vi "Power-HWP test.vi"(8 "Error In":errorcluster, 10 "Cluster In":T2={"Position"=0.0, "Is.Enabled?"=FALSE, "Is.Connected?"=FALSE, "Device SN"="55151324", "AccelerationMaximum"=10.0, "VelocityMaximum"=10.0, "Acceleration"=10.0, "Velocity"=10.0, "waitTimeout (ms)"=10000, "Model"=enum."None", "Is.Homed?"=FALSE, "MOVE"=FALSE}) -> (0 "Error Out":errorcluster)   [LabVIEW 2018]
uses:
  Hardware Mfg/Thorlabs Translation Stages/Controls/Translation Stage Cluster.ctl
  General/Controls/Translation Stage Types.ctl
  C:/Project/SerialSectionOCT/SerialSectOCT/Labview Software/Thorlabs.MotionControl.Controls.dll
  Thorlabs.MotionControl.Controls.dll
  KnifeEdgeTestClt.ctl
  Hardware Mfg/Thorlabs Cage Rotation/refnum control.ctl
  General/Controls/Set Get Controls.ctl
  Hardware Mfg/Thorlabs Translation Stages/Controls/Motion Translation Module Control2.ctl
  <vilib>/DAQmx/read.llb/DAQmx Read (Analog 1D Wfm NChan NSamp).vi
  <vilib>/DAQmx/create/channels.llb/DAQmx Create Channel (AI-Voltage-Basic).vi
  <vilib>/DAQmx/configure/timing.llb/DAQmx Timing (Sample Clock).vi
  <vilib>/DAQmx/configure/task.llb/DAQmx Configure Logging (TDMS).vi
  <vilib>/DAQmx/configure/trigger.llb/DAQmx Start Trigger (Digital Edge).vi
  <vilib>/DAQmx/configure/trigger.llb/DAQmx Start Trigger (Time).vi
  <vilib>/DAQmx/configure/trigger.llb/DAQmx Start Trigger (Analog Edge).vi
  <vilib>/DAQmx/miscellaneous.llb/DAQmx Fill In Error Info.vi
  <resource>/objmgr/daqmx.rc
panel:
  in  "Trigger Type":T1(tab)
  in  "Digital Start Trigger Edge":i32(ring)=10280 caption="Edge" items=["Rising"=10280, "Falling"=10171]
  in  "Digital Start Trigger Source":tag="/Dev1/PFI0" caption="Source"
  in  "Digital Pause Trigger Pause When":i32(ring)=10192 caption="Pause When" items=["High"=10192, "Low"=10214]
  in  "Digital Pause Trigger Source":tag="/Dev1/PFI0" caption="Source"
  in  "Analog Start Trigger Level":dbl caption="Level" format="%0.2f"
  in  "Analog Start Trigger Hysteresis":dbl caption="Hysteresis" format="%.2f"
  in  "Analog Start Trigger Slope":i32(ring)=10280 caption="Slope" items=["Rising"=10280, "Falling"=10171]
  in  "Analog Start Trigger Source":string="APFI0" caption="Source"
  in  "Analog Pause Trigger Source":string="APFI0" caption="Source"
  in  "Analog Pause Trigger Pause When":i32(ring)=10093 caption="Pause When" items=["Above Level"=10093, "Below Level"=10107]
  in  "Analog Pause Trigger Level":dbl caption="Level" format="%.2f"
  in  "When":timestamp
  in  "Select Time\nManually":bool
  in  "Number of Samples":i32=100
  in  "TDMS File Path":path
  in  "Sample Rate":dbl=1000.0
  in  "Sample Clock Source":tag="OnboardClock"
  in  "Terminal Configuration":i32(ring)=-1 items=["default"=-1, "RSE"=10083, "NRSE"=10078, "Differential"=10106, "Pseudodifferential"=12529]
  in  "Max Voltage":dbl=5.0
  in  "Min Voltage":dbl=-5.0
  in  "Physical Channel":tag="Dev1/ai0"
  out "Actual Sample Rate":dbl=1000.0 format="%0.2f"
  in  "Logging Mode":i32(ring)=10231 items=["Off"=10231, "Log and Read"=15842]
  in  "LTS Reference":refnum<k24>(container)
  out "Power":dbl
  in  "Start":dbl
  in  "Stop":dbl=90.0
  in  "step size":dbl=1.0
  out "Wavelength [nm] 2":dbl caption="Wavelength"
  out "Avg. Time  [sec.]":dbl caption="Average Time"
  out "Average Count 2":i32 caption="Average Time"
  in  "Avg. Time (0.0) [sec.]":dbl=1.5 caption="Average Time (0.0)" min=0.1 max=5.0 step=0.1
  in  "Wavelength [nm]":dbl=840.0 caption="Wavelength (0.0)"
  in  "Average Count":i32=10 min=1 step=1
  in  "path":path=path "C:/Users/BOAS-USER/Documents/Data/210615_2P_power_calibration/test.csv"
  # "To enable triggers, select a tab above, and configure the settings.\n\nNot all hardware supports all trigger types. Refer to your device documentation for more information."
  # "This trigger type is not supported in continuous sample timing. \n\nRefer to your device documentation for more information on which triggers are supported."
  # "This trigger type is not supported in continuous sample timing. \n\nRefer to your device documentation for more information on which triggers are supported."
  # "If time is not manually set, task will begin after 10 seconds"
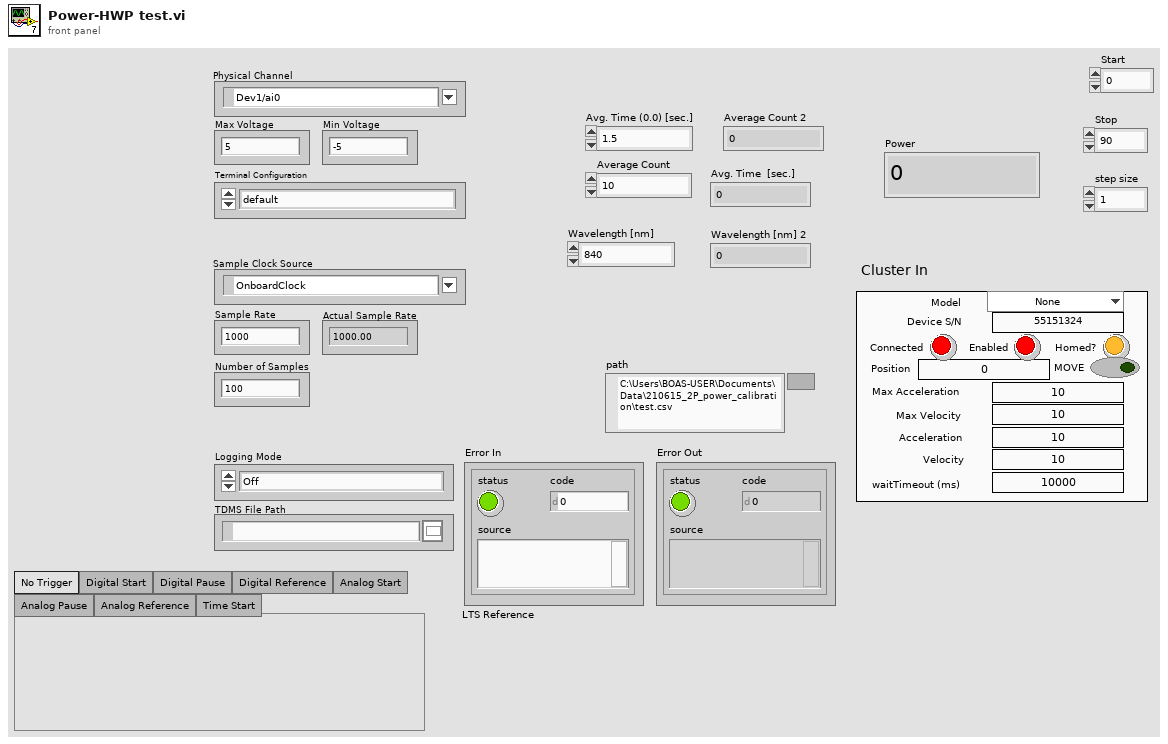
[diagram p1: front panel]
types:
  T1 = enum32{"No Trigger", "Digital Start", "Digital Pause", "Digital Reference", "Analog Start", "Analog Pause", "Analog Reference", "Time Start"}
  T2 = typedef "Translation Stage Cluster.ctl" = cluster{"Position":dbl, "Is.Enabled?":bool, "Is.Connected?":bool, "Device SN":string, "AccelerationMaximum":dbl, "VelocityMaximum":dbl, "Acceleration":dbl, "Velocity":dbl, "waitTimeout (ms)":i32, "Model":T3, "Is.Homed?":bool, "MOVE":bool}
  T3 = typedef "Translation Stage Types.ctl" = enum16{"None", "Thorlabs LTS", "Thorlabs MLJ"}
  T4 = typedef "KnifeEdgeTestClt.ctl" = enum16{"Init Power meter", "Init Table stages", "Go stage home", "Move stage", "Power meter thorlabs", "Uninit", "Generate steps", "Power meter PDA50B2", "Init PDA50B2"}
  T5 = typedef "refnum control.ctl" = enum16{"Get", "Init"}
  T6 = typedef "Motion Translation Module Control2.ctl" = enum16{"Init", "Home", "Status", "Velocity/Accel", "Position", "Jog", "Stop", "Uninit", "Enable", "Disable"}
  T7 = typedef "Set Get Controls.ctl" = enum16{"Set", "Get"}
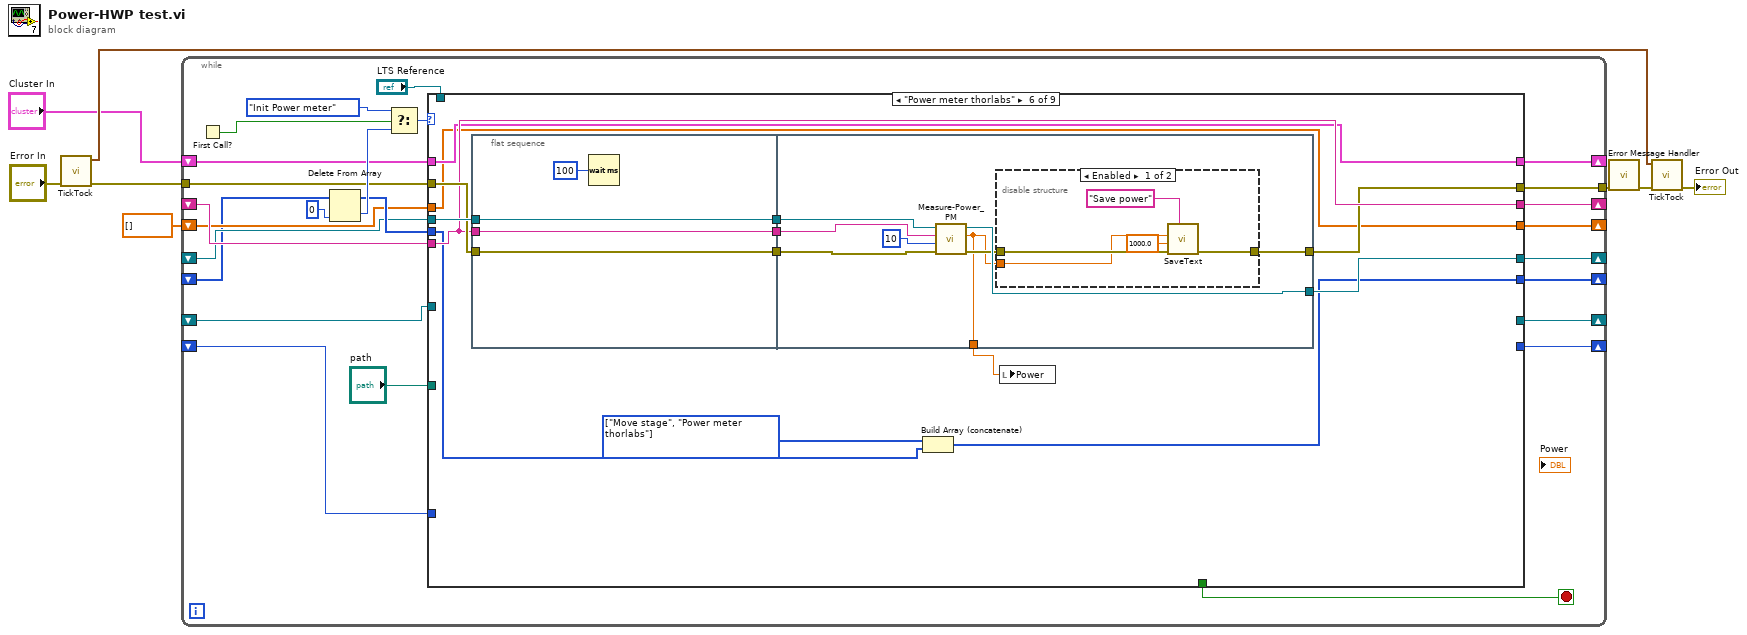
[diagram p0: block diagram]
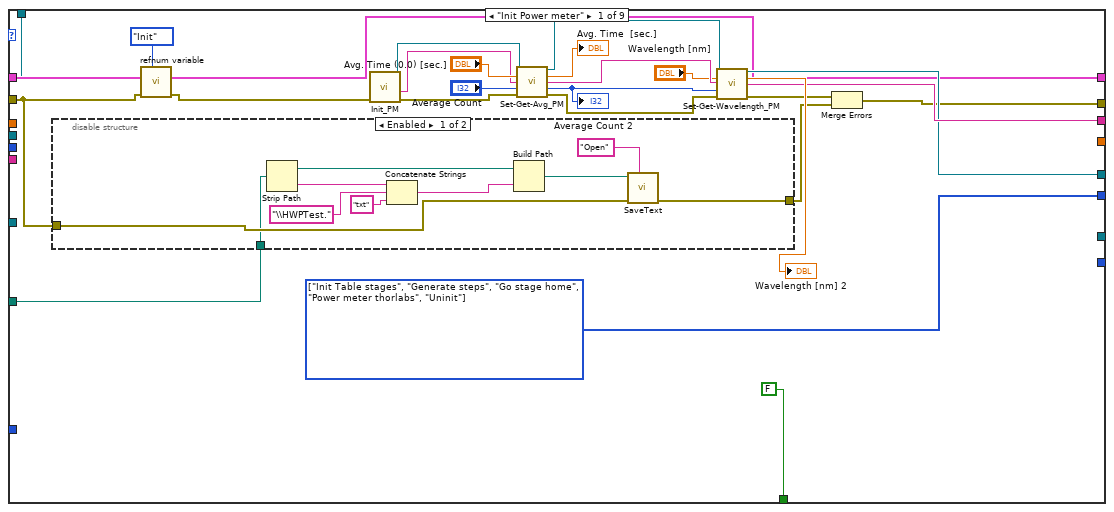
[diagram p2: hidden frame]
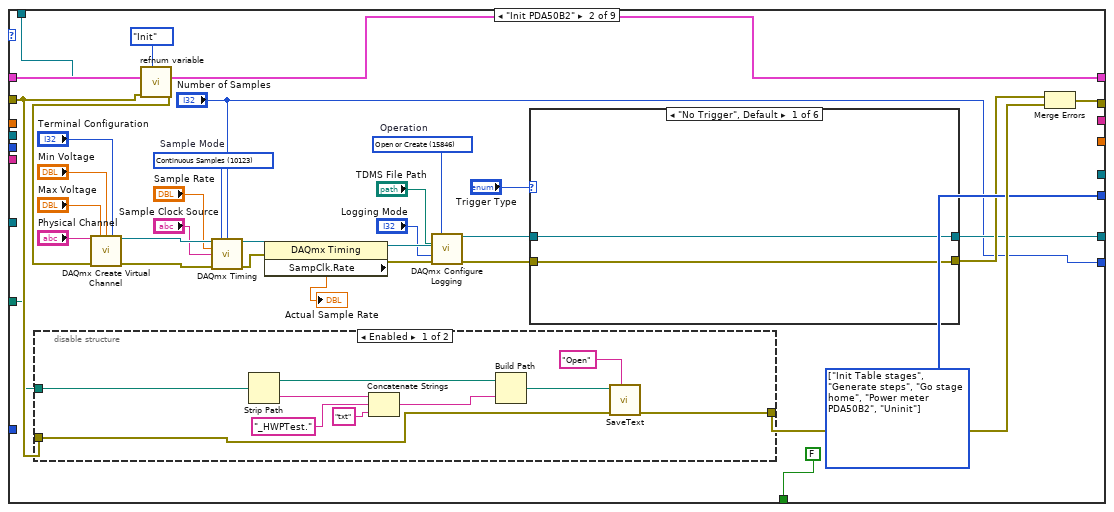
[diagram p4: hidden frame]
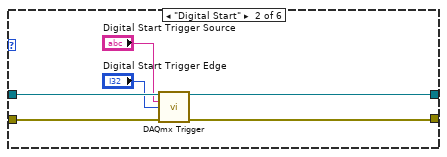
[diagram p5: hidden frame]
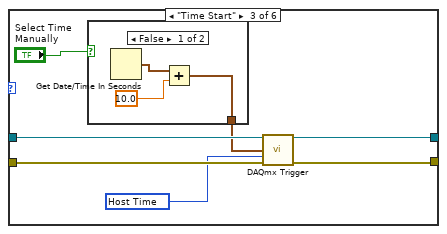
[diagram p6: hidden frame]
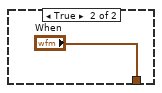
[diagram p7: hidden frame]
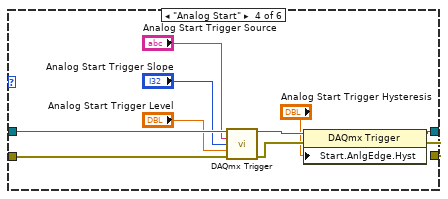
[diagram p8: hidden frame]
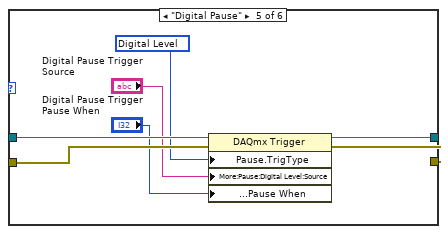
[diagram p9: hidden frame]
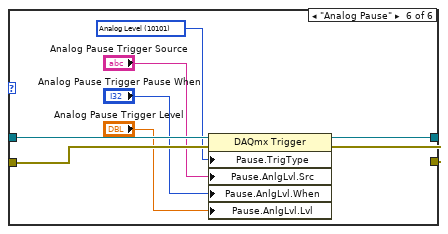
[diagram p10: hidden frame]
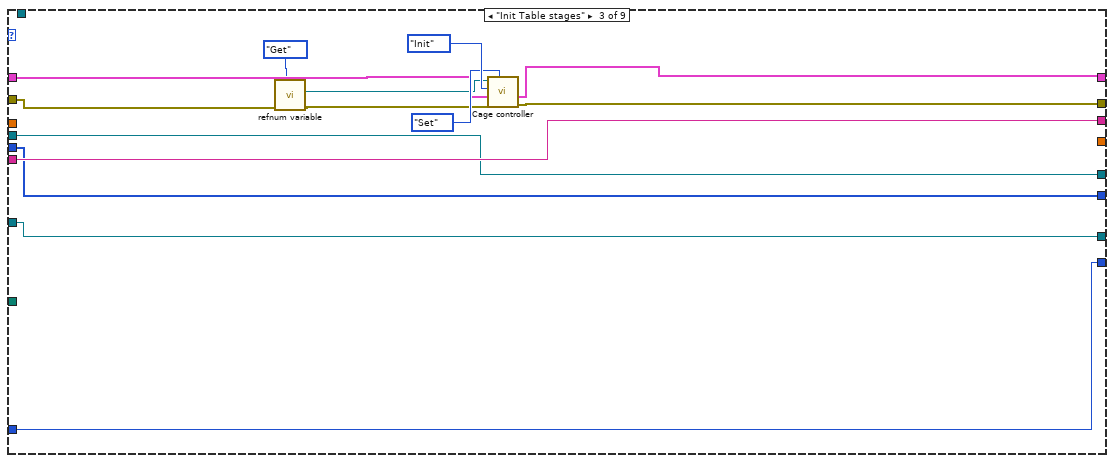
[diagram p12: hidden frame]
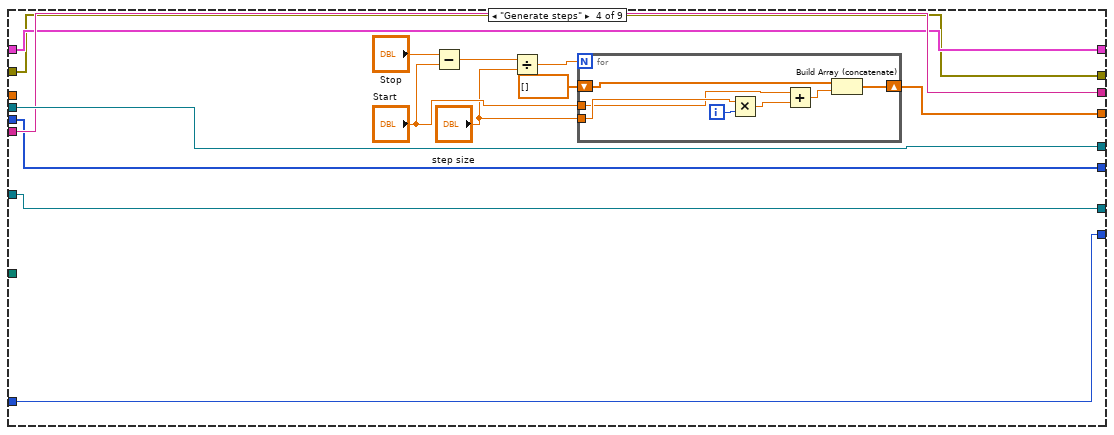
[diagram p13: hidden frame]
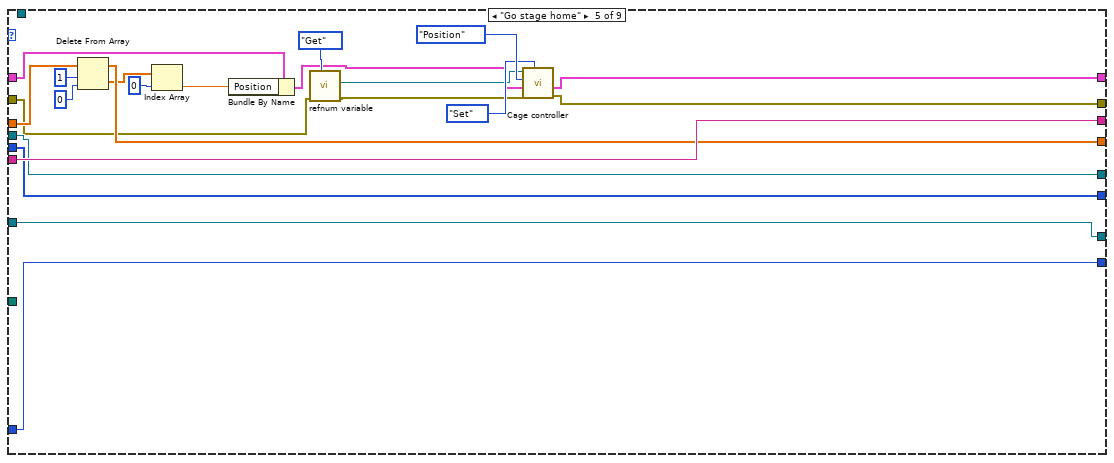
[diagram p14: hidden frame]
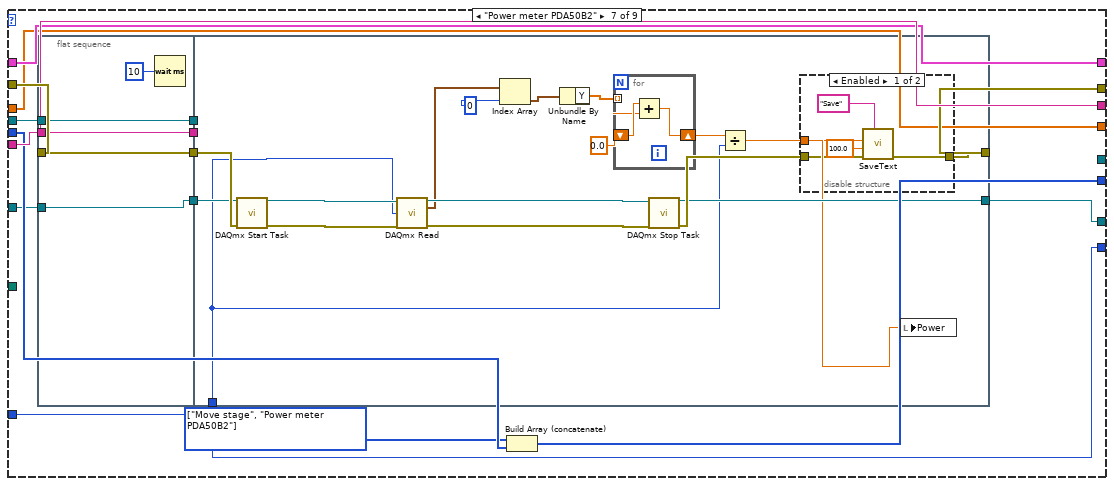
[diagram p16: hidden frame]
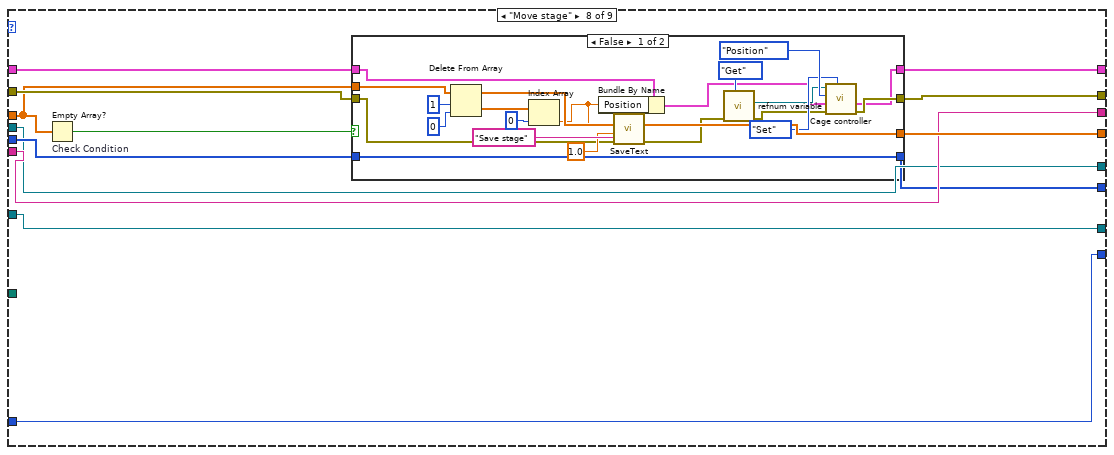
[diagram p18: hidden frame]
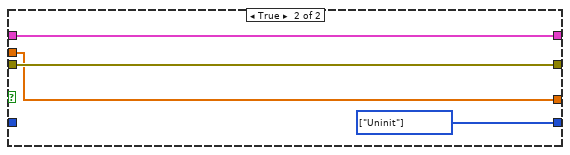
[diagram p19: hidden frame]
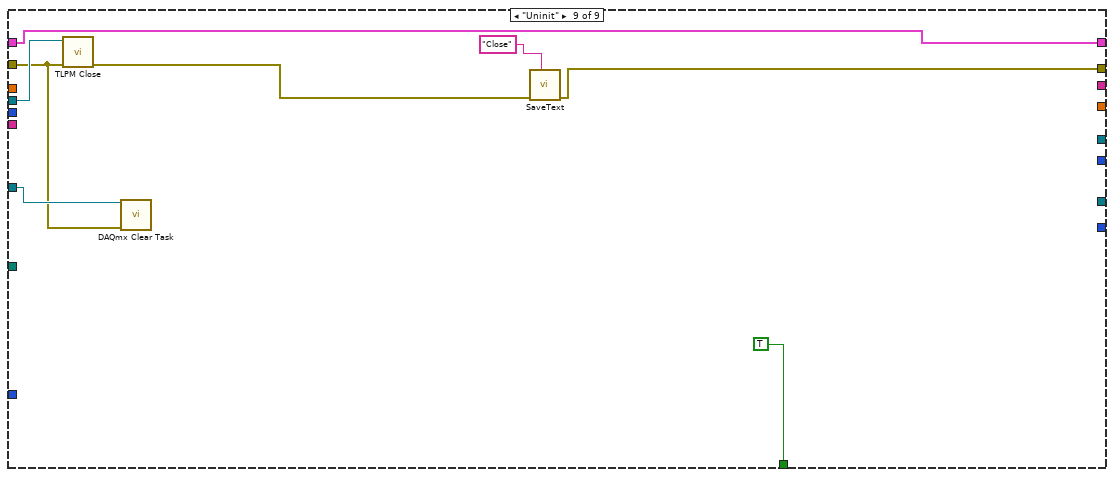
[diagram p20: hidden frame]
diagram:
  n1 = call "TickTock.vi"("Error In"="Error In") -> ("Error Out"=w6:errorcluster, "Current Time (Out)"=w4:timestamp)  [unwired: 8 in, 1 out]
  n2 = while {
    tunnel: w6 -> [w29]
    tunnel: [w28] -> w8
    shift-right: [w27] -> _
    shift-left: _ -> [w25]
    shift-right: [w26] -> _
    shift-left: _ -> [w24]
    shift-right: [w21] -> _
    shift-left: "Cluster In" -> [w22]
    shift-right: [w20] -> _
    shift-left: dbl[] [] -> [w19]
    shift-right: [w18] -> _
    shift-left: _ -> [w17]
    shift-right: [w14] -> _
    shift-left: _ -> [w11]
    shift-right: [w13] -> _
    shift-left: _ -> [w12]
    stop <- w16 stop-if-true
    n3 = First Call?() -> (First Call?: T/F=w15:bool)
    n4 = Delete From Array(array=w17, index=0) -> (deleted portion=w32:T4, array with subset deleted=w31:T4[])  [unwired: 1 in]
    n5 = Select(t=KnifeEdgeTestClt."Init Power meter", s=w15, f=w32) -> (s? t:f=w33:T4)
    n6 = case shown="\"Power meter thorlabs\"" w33 {
      tunnel: [w36 w95 w167 w175 w203 w215 w250 w295 _] -> w18
      tunnel: w31 -> [_ _ w167 w175 w203 w216 w251 w302 _]
      tunnel: [_ _ _ w171 w208 w217 w252 w304 _] -> w20
      tunnel: w29 -> [w39 w97 w160 w170 w196 w225 w259 w301 w330]
      tunnel: [w43 w100 w166 w170 w195 w222 w257 w300 w334] -> w28
      tunnel: [w46 _ w169 w182 w212 w223 w258 w299 _] -> w27
      tunnel: [w45 _ w168 w183 w202 w224 _ w298 _] -> w26
      tunnel: w25 -> [_ _ w169 w182 w212 w223 w258 w299 _]
      tunnel: w24 -> [_ _ w168 w183 w202 w226 w260 w298 w337]
      tunnel: w22 -> [w41 w99 w163 w181 w207 w218 w253 w297 w336]
      tunnel: [w41 w99 w162 w181 w193 w218 w253 w296 w336] -> w21
      tunnel: w19 -> [_ _ _ _ w211 w217 w252 w294 _]
      tunnel: [FALSE FALSE _ _ _ _ _ _ TRUE] -> w16
      tunnel: [_ w72 w157 w173 w192 _ w246 w293 _] -> w14
      tunnel: [_ "Number of Samples" w156 w172 w191 _ w245 w292 _] -> w13
      tunnel: w12 -> [_ _ w156 w172 w191 _ w245 w292 _]
      tunnel: w11 -> [_ _ w157 w173 w192 _ w247 w293 w332]
      tunnel: "path" -> [w35 w70 _ _ _ _ _ _ _]
      tunnel: "LTS Reference" -> [w34 w69 _ _ _ _ _ _ _]
      frame "Init Power meter" {
        w36 = T4[] [enum."Init Table stages", enum."Generate steps", enum."Go stage home", enum."Power meter thorlabs", enum."Uninit"] items=["Init Power meter", "Init Table stages", "Go stage home", "Move stage", "Power meter thorlabs", "Uninit", "Generate steps", "Power meter PDA50B2", "Init PDA50B2"]
        n7 = disable-structure shown="Enabled" {
          disable-tunnel: w39 -> [w64 _]
          disable-tunnel: [w63 _] -> w44
          disable-tunnel: w35 -> [w59 _]
          frame Enabled {
            n8 = Strip Path(path=w59) -> (stripped path=w61:path, name=w66:string)
            n9 = Concatenate Strings(w66, "\\HWPTest." ("string"), "txt" ("string")) -> (w62:string)
            n10 = Build Path(base path=w61, name or relative path=w62) -> (appended path=w60:path)
            n11 = call "SaveText.vi"("action"="Open", "error in"=w64, "file path (use dialog)"=w60) -> ("error out"=w63:errorcluster)  [unwired: 8 in]
          }
          frame Disabled {
          }
        }
        n12 = call "refnum variable.vi"("action"=refnum_control."Init", "error in (no error)"=w39, "reference in"=w34) -> ("error out"=w38:errorcluster)  [unwired: 7 in, 1 out]
        n13 = call "Init_PM.vi"("error in (no error)"=w38) -> ("error out"=w47:errorcluster, "Sensor Name"=w48:string, "instrument handle out"=w49:refnum<visa-resource-name>)  [unwired: 8 in]
        n14 = call "Set-Get-Avg_PM.vi"("instrument handle"=w49, "Average Time (0.0)"="Avg. Time (0.0) [sec.]", "Sensor"=w48, "Average Count"="Average Count", "error in (no error)"=w47) -> ("instrument handle out"=w56:refnum<visa-resource-name>, "Average Time"=→"Avg. Time  [sec.]":dbl, "Sensor 2"=w54:string, "Average Count"=w53:i32, "error out"=w57:errorcluster)  [unwired: 6 in]
        "Average Count 2" <- w53
        n15 = call "Set-Get-Wavelength_PM.vi"("instrument handle"=w56, "Wavelength"="Wavelength [nm]", "Sensor Name"=w54, "Average Count"=w53, "error in (no error)"=w57) -> ("instrument handle out"=w45:refnum<visa-resource-name>, "Wavelength"=→"Wavelength [nm] 2":dbl, "Sensor Name 2"=w46:string, "error out"=w42:errorcluster)  [unwired: 6 in, 1 out]
        n16 = Merge Errors(w42, w44) -> (w43:errorcluster)
      }
      frame "Init PDA50B2" {
        w87 = 15846 items=["Open"=10437, "Open or Create"=15846, "Create or Replace"=15847, "Create"=15848]  # Operation
        w92 = 10123 items=["Finite Samples"=10178, "Continuous Samples"=10123, "Hardware Timed Single Point"=12522]  # Sample Mode
        w95 = T4[] [enum."Init Table stages", enum."Generate steps", enum."Go stage home", enum."Power meter PDA50B2", enum."Uninit"] items=["Init Power meter", "Init Table stages", "Go stage home", "Move stage", "Power meter thorlabs", "Uninit", "Generate steps", "Power meter PDA50B2", "Init PDA50B2"]
        n17 = disable-structure shown="Enabled" {
          disable-tunnel: w97 -> [w151 _]
          disable-tunnel: [w150 _] -> w101
          disable-tunnel: w70 -> [w146 _]
          frame Enabled {
            n18 = Strip Path(path=w146) -> (stripped path=w148:path, name=w153:string)
            n19 = Concatenate Strings(w153, "_HWPTest." ("string"), "txt" ("string")) -> (w149:string)
            n20 = Build Path(base path=w148, name or relative path=w149) -> (appended path=w147:path)
            n21 = call "SaveText.vi"("action"="Open", "error in"=w151, "file path (use dialog)"=w147) -> ("error out"=w150:errorcluster)  [unwired: 8 in]
          }
          frame Disabled {
          }
        }
        n22 = call "refnum variable.vi"("action"=refnum_control."Init", "error in (no error)"=w97, "reference in"=w69) -> ("error out"=w73:errorcluster)  [unwired: 7 in, 1 out]
        n23 = call-poly <vilib>:"DAQmx Create Virtual Channel.vi"("maximum value"="Max Voltage", "minimum value"="Min Voltage", "input terminal configuration"="Terminal Configuration", "physical channels"="Physical Channel", "error in"=w73) -> ("task out"=w90:refnum<k21>, "error out"=w91:errorcluster)  [unwired: 9 in]
        n24 = call-poly <vilib>:"DAQmx Timing.vi"("task/channels in"=w90, "sample mode"=w92, "samples per channel"="Number of Samples", "rate"="Sample Rate", "source"="Sample Clock Source", "error in"=w91) -> ("task out"=w94:refnum<k21>, "error out"=w93:errorcluster)  [unwired: 8 in]
        n25 = property class="DAQmx Timing"(reference=w94, error in=w93) -> (reference out=w89:refnum<k21>, error out=w88:errorcluster, "SampClk.Rate"=→"Actual Sample Rate":dbl)
        n26 = call-poly <vilib>:"DAQmx Configure Logging.vi"("task/channels in"=w89, "operation"=w87, "file path"="TDMS File Path", "logging mode"="Logging Mode", "error in"=w88) -> ("task out"=w76:refnum<k21>, "error out"=w75:errorcluster)  [unwired: 9 in]
        n27 = case shown="\"No Trigger\", Default" "Trigger Type" {
          tunnel: w76 -> [w103 w109 w116 w130 w137 w145]
          tunnel: w75 -> [w102 w108 w115 w129 w134 w142]
          tunnel: [w103 w107 w114 w127 w136 w144] -> w72
          tunnel: [w102 w106 w113 w126 w135 w143] -> w74
          frame "No Trigger", Default {
          }
          frame "Digital Start" {
            n28 = call-poly <vilib>:"DAQmx Trigger.vi"("task/channels in"=w109, "source"="Digital Start Trigger Source", "edge"="Digital Start Trigger Edge", "error in"=w108) -> ("task out"=w107:refnum<k21>, "error out"=w106:errorcluster)  [unwired: 10 in]
          }
          frame "Time Start" {
            w112 = 16126 items=["Host Time"=16126, "I/O Device Time"=16127] ("timescale")
            n29 = case shown="False" "Select Time\nManually" {
              tunnel: [w117 "When"] -> w110
              frame False {
                n30 = Get Date/Time In Seconds() -> (seconds since 1Jan1904=w119:timestamp)
                n31 = Add(x=w119, y=10.0) -> (x+y=w117:timestamp)
              }
              frame True {
              }
            }
            n32 = call-poly <vilib>:"DAQmx Trigger.vi"("task/channels in"=w116, "when"=w110, "timescale"=w112, "error in"=w115) -> ("task out"=w114:refnum<k21>, "error out"=w113:errorcluster)  [unwired: 10 in]
          }
          frame "Analog Start" {
            n33 = call-poly <vilib>:"DAQmx Trigger.vi"("task/channels in"=w130, "source"="Analog Start Trigger Source", "slope"="Analog Start Trigger Slope", "level"="Analog Start Trigger Level", "error in"=w129) -> ("task out"=w125:refnum<k21>, "error out"=w124:errorcluster)  [unwired: 9 in]
            n34 = property class="DAQmx Trigger"(reference=w125, error in=w124, "Start.AnlgEdge.Hyst"="Analog Start Trigger Hysteresis") -> (reference out=w127:refnum<k21>, error out=w126:errorcluster)
          }
          frame "Digital Pause" {
            w133 = 10152 items=["Analog Level"=10101, "Analog Window"=10103, "Digital Level"=10152, "Digital Pattern"=10398, "None"=10230] ("Pause.TrigType")
            n35 = property class="DAQmx Trigger"(reference=w137, error in=w134, "Pause.TrigType"=w133, "More:Pause:Digital Level:Source"="Digital Pause Trigger Source", "More:Pause:Digital Level:Pause When"="Digital Pause Trigger Pause When") -> (reference out=w136:refnum<k21>, error out=w135:errorcluster)
          }
          frame "Analog Pause" {
            w141 = 10101 items=["Analog Level"=10101, "Analog Window"=10103, "Digital Level"=10152, "Digital Pattern"=10398, "None"=10230] ("Pause.TrigType")
            n36 = property class="DAQmx Trigger"(reference=w145, error in=w142, "Pause.TrigType"=w141, "Pause.AnlgLvl.Src"="Analog Pause Trigger Source", "Pause.AnlgLvl.When"="Analog Pause Trigger Pause When", "Pause.AnlgLvl.Lvl"="Analog Pause Trigger Level") -> (reference out=w144:refnum<k21>, error out=w143:errorcluster)
          }
        }
        n37 = Merge Errors(w74, w101) -> (w100:errorcluster)
      }
      frame "Init Table stages" {
        n38 = call "refnum variable.vi"("action"=refnum_control."Get", "error in (no error)"=w160) -> ("error out"=w159:errorcluster, "reference in 2"=w158:refnum<k24>)  [unwired: 8 in]
        n39 = call "Cage controller.vi"("Set/Get"=Set_Get_Controls."Set", "error in (no error)"=w159, "Cluster In"=w163, "Action"=Motion_Translation_Module_Control2."Init", "reference in"=w158) -> ("error out"=w166:errorcluster, "Cluster out"=w162:T2)  [unwired: 4 in, 1 out]
      }
      frame "Generate steps" {
        n40 = Subtract(x="Stop", y="Start") -> (x-y=w179:dbl)
        n41 = Divide(x=w179, y="step size") -> (x/y=w178:dbl)
        n42 = for {
          N: w178 -> [_]
          tunnel: "Start" -> [w188]
          tunnel: "step size" -> [w189]
          shift-right: [w185] -> w171
          shift-left: dbl[] [] -> [w184]
          i -> [w190]
          n43 = Multiply(x=w189, y=w190) -> (x*y=w187:dbl)
          n44 = Add(x=w188, y=w187) -> (x+y=w186:dbl)
          n45 = Build Array (concatenate)(w184, w186) -> (w185:dbl[])
        }
      }
      frame "Go stage home" {
        n46 = Delete From Array(array=w211, length=1, index=0) -> (deleted portion=w206:dbl[], array with subset deleted=w208:dbl[])
        n47 = Index Array(array=w206, index=0) -> (element=w204:dbl)
        n48 = Bundle By Name(cluster=w207, "Position"=w204) -> (w194:T2)
        n49 = call "refnum variable.vi"("action"=refnum_control."Get", "error in (no error)"=w196) -> ("error out"=w198:errorcluster, "reference in 2"=w197:refnum<k24>)  [unwired: 8 in]
        n50 = call "Cage controller.vi"("Set/Get"=Set_Get_Controls."Set", "error in (no error)"=w198, "Cluster In"=w194, "Action"=Motion_Translation_Module_Control2."Position", "reference in"=w197) -> ("error out"=w195:errorcluster, "Cluster out"=w193:T2)  [unwired: 4 in, 1 out]
      }
      frame "Power meter thorlabs" {
        w214 = T4[] [enum."Move stage", enum."Power meter thorlabs"] items=["Init Power meter", "Init Table stages", "Go stage home", "Move stage", "Power meter thorlabs", "Uninit", "Generate steps", "Power meter PDA50B2", "Init PDA50B2"]
        n51 = flat-sequence {
          tunnel: w223 -> [w228]
          tunnel: w225 -> [w229]
          tunnel: w226 -> [w230]
          tunnel: [w230] -> w221
          tunnel: [w229] -> w220
          tunnel: [w228] -> w219
          tunnel: [w236] -> w224
          tunnel: [w234] -> w222
          tunnel: w221 -> [w238]
          tunnel: w220 -> [w237]
          tunnel: w219 -> [w235]
          tunnel: [w231] -> w213
          frame #0 {
            n52 = Wait (ms)(milliseconds to wait=u32 100) -> ()  [unwired: 1 out]
          }
          frame #1 {
            n53 = call "Measure-Power_PM.vi"("error in (no error)"=w237, "Numeric"=10, "Sensor"=w235, "instrument handle"=w238) -> ("error out"=w232:errorcluster, "Power"=w231:dbl, "instrument handle out"=w236:refnum<visa-resource-name>)  [unwired: 5 in]
            n54 = disable-structure shown="Enabled" {
              disable-tunnel: [w243 w244] -> w234
              disable-tunnel: w232 -> [w242 w244]
              disable-tunnel: w231 -> [w240 _]
              frame Enabled {
                n55 = call "SaveText.vi"("action"="Save power", "error in"=w242, "GAIN"=sgl 1000.0, "data in"=w240) -> ("error out"=w243:errorcluster)  [unwired: 7 in]
              }
              frame Disabled {
              }
            }
          }
        }
        n56 = Build Array (concatenate)(w214, w216) -> (w215:T4[])
        n57 = local write "Power"(w213) -> ()
      }
      frame "Power meter PDA50B2" {
        w249 = T4[] [enum."Move stage", enum."Power meter PDA50B2"] items=["Init Power meter", "Init Table stages", "Go stage home", "Move stage", "Power meter thorlabs", "Uninit", "Generate steps", "Power meter PDA50B2", "Init PDA50B2"]
        n58 = flat-sequence {
          tunnel: w258 -> [w263]
          tunnel: w259 -> [w264]
          tunnel: w260 -> [w265]
          tunnel: [w265] -> w256
          tunnel: [w264] -> w255
          tunnel: [w263] -> w254
          tunnel: w247 -> [w261]
          tunnel: [w261] -> w248
          tunnel: [w282] -> w257
          tunnel: w256 -> [_]
          tunnel: w255 -> [w277]
          tunnel: w254 -> [_]
          tunnel: w245 -> [w271]
          tunnel: w248 -> [w275]
          tunnel: [w274] -> w246
          frame #0 {
            n59 = Wait (ms)(milliseconds to wait=u32 10) -> ()  [unwired: 1 out]
          }
          frame #1 {
            n60 = call <vilib>:"DAQmx Start Task.vi"("task/channels in"=w275, "error in"=w277) -> ("task out"=w281:refnum<k21>, "error out"=w280:errorcluster)  [unwired: 12 in]
            n61 = call-poly <vilib>:"DAQmx Read.vi"("task/channels in"=w281, "number of samples per channel"=w271, "error in"=w280) -> ("task out"=w279:refnum<k21>, "data"=w270:waveform(dbl)[], "error out"=w278:errorcluster)  [unwired: 10 in]
            n62 = Index Array(array=w270, index=0) -> (element=w268:waveform(dbl))
            n63 = Unbundle By Name(w268) -> ("Y"=w267:dbl[])
            n64 = for {
              shift-right: [w284] -> w272
              shift-left: 0.0 -> [w285]
              tunnel: w267 -> [w283] mode=indexing
              n65 = Add(x=w285, y=w283) -> (x+y=w284:dbl)
            }
            n66 = call <vilib>:"DAQmx Stop Task.vi"("task/channels in"=w279, "error in"=w278) -> ("task out"=w274:refnum<k21>, "error out"=w276:errorcluster)  [unwired: 12 in]
            n67 = Divide(x=w272, y=w271) -> (x/y=w266:dbl)
            n68 = disable-structure shown="Enabled" {
              disable-tunnel: [w290 w291] -> w282
              disable-tunnel: w276 -> [w289 w291]
              disable-tunnel: w266 -> [w287 _]
              frame Enabled {
                n69 = call "SaveText.vi"("action"="Save", "error in"=w289, "GAIN"=sgl 100.0, "data in"=w287) -> ("error out"=w290:errorcluster)  [unwired: 7 in]
              }
              frame Disabled {
              }
            }
            n70 = local write "Power"(w266) -> ()
          }
        }
        n71 = Build Array (concatenate)(w249, w251) -> (w250:T4[])
      }
      frame "Move stage" {
        n72 = Empty Array? "Check Condition"(array=w294) -> (empty?=w303:bool)
        n73 = case shown="False" w303 {
          tunnel: [w319 w328] -> w304
          tunnel: w302 -> [w318 _]
          tunnel: [w318 w326] -> w295
          tunnel: w301 -> [w306 w329]
          tunnel: [w312 w329] -> w300
          tunnel: w297 -> [w321 w327]
          tunnel: [w311 w327] -> w296
          tunnel: w294 -> [w320 w328]
          frame False {
            n74 = Delete From Array(array=w320, length=1, index=0) -> (deleted portion=w323:dbl[], array with subset deleted=w319:dbl[])
            n75 = Index Array(array=w323, index=0) -> (element=w305:dbl)
            n76 = Bundle By Name(cluster=w321, "Position"=w305) -> (w310:T2)
            n77 = call "SaveText.vi"("action"="Save stage", "error in"=w306, "GAIN"=sgl 1.0, "data in"=w305) -> ("error out"=w307:errorcluster)  [unwired: 7 in]
            n78 = call "refnum variable.vi"("action"=refnum_control."Get", "error in (no error)"=w307) -> ("error out"=w314:errorcluster, "reference in 2"=w313:refnum<k24>)  [unwired: 8 in]
            n79 = call "Cage controller.vi"("Set/Get"=Set_Get_Controls."Set", "error in (no error)"=w314, "Cluster In"=w310, "Action"=Motion_Translation_Module_Control2."Position", "reference in"=w313) -> ("error out"=w312:errorcluster, "Cluster out"=w311:T2)  [unwired: 4 in, 1 out]
          }
          frame True {
            w326 = T4[] [enum."Uninit"] items=["Init Power meter", "Init Table stages", "Go stage home", "Move stage", "Power meter thorlabs", "Uninit", "Generate steps", "Power meter PDA50B2", "Init PDA50B2"]
          }
        }
      }
      frame "Uninit" {
        n80 = call "TLPM Close.vi"("error in (no error)"=w330, "instrument handle"=w337) -> ("error out"=w331:errorcluster)  [unwired: 9 in]
        n81 = call <vilib>:"DAQmx Clear Task.vi"("task in"=w332, "error in"=w330) -> ()  [unwired: 13 in, 1 out]
        n82 = call "SaveText.vi"("action"="Close", "error in"=w331) -> ("error out"=w334:errorcluster)  [unwired: 9 in]
      }
    }
  }
  n83 = call "Error Message Handler.vi"("Error In"=w8) -> ("Error Out"=w3:errorcluster)  [unwired: 9 in, 1 out]
  n84 = call "TickTock.vi"("Error In"=w3, "Current Time (In)"=w4) -> ("Error Out"=→"Error Out":errorcluster)  [unwired: 7 in, 2 out]
